vi "Translate Data.vi"(8 "error in":errorcluster, 10 "BufferIn":string, 11 "M in":refnum<class "M.lvclass">) -> (0 "error out":errorcluster, 2 "DataOut":refnum<class "Data.lvclass">, 3 "M out":refnum<class "M.lvclass">)   [LabVIEW 2015, in "Alicat.lvlib" / "M.lvclass"]
doc: "VI used to translate the data buffer to something meaningful (implementation dependent). This VI must be overridden."
uses:
  M.lvclass
  Reusable/Data/Data.lvclass
  Data/MC/AlicatMCData.lvclass
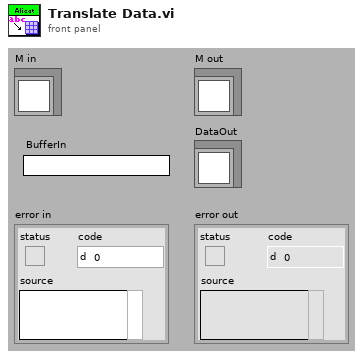
[diagram p1: front panel]
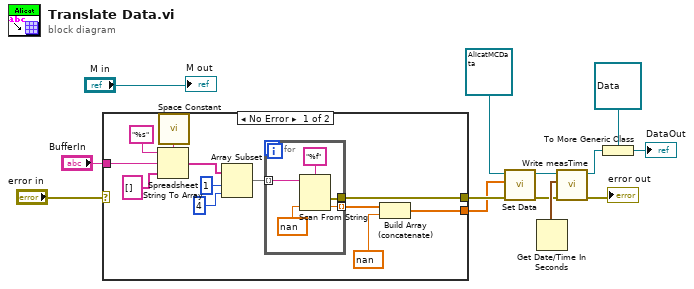
[diagram p0: block diagram]
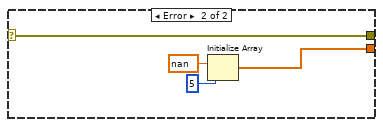
[diagram p2: hidden frame]
diagram:
  n1 = case shown="No Error" "error in" {
    selector: "error in" -> [_ w34]
    tunnel: "BufferIn" -> [w22 _]
    tunnel: [w15 w32] -> w4
    tunnel: [w21 w34] -> w10
    frame No Error {
      n2 = call <vilib>:"Space Constant.vi"() -> ("String"=w24:string)
      n3 = Spreadsheet String To Array(delimiter (Tab)=w24, format string="%s", spreadsheet string=w22, array type (2D Dbl)=string[] []) -> (array=w20:string[])
      n4 = Array Subset(array=w20, index=1, length=4) -> (w18:string[])
      n5 = for {
        tunnel: w18 -> [w30] mode=indexing
        tunnel: [w27] -> w17 mode=indexing
        tunnel: [w26] -> w21
        n6 = Scan From String(format string="%f", input string=w30, default 1=sgl nan ("default value 1")) -> (error out=w26:errorcluster, output 1=w27:sgl)  [unwired: 2 in, 2 out]
      }
      n7 = Build Array (concatenate)(w17, sgl nan ("default value 1")) -> (w15:sgl[])
    }
    frame Error {
      n8 = Initialize Array(sgl nan ("element"), 5 ("dimension size")) -> (w32:sgl[])
    }
  }
  n9 = call "Set Data.vi"("error in"=w10, "DataIn"=w4, "AlicatMData in"=refnum<class "AlicatMCData.lvclass"> refnum ("AlicatMCData.lvclass")) -> ("error out"=w9:errorcluster, "AlicatMData out"=w12:refnum<class "AlicatMCData.lvclass">)  [unwired: 7 in]
  n10 = Get Date/Time In Seconds() -> (seconds since 1Jan1904=w11:timestamp)
  n11 = call "Write measTime.vi"("error in (no error)"=w9, "measTime"=w11, "Data in"=w12) -> ("error out"=→"error out":errorcluster, "Data out"=w3:refnum<class "AlicatMCData.lvclass">)  [unwired: 7 in]
  n12 = To More Generic Class(target class=refnum<class "Data.lvclass"> refnum ("DataOut"), reference=w3) -> (generic class reference=→"DataOut":refnum<class "Data.lvclass">)
  "M out" <- "M in"
